vi "Terminal_Gear_System_Dispaly.vi"   [LabVIEW 2014]
types:
  T1 = cluster{"润滑油流量":u16, "油箱润滑油液位":u16, "油箱温度":u16, "冷却装置工作状态":u16, "供油压力":u16, "过滤器压差":u16, "油箱液位":u16, "供油油温":u16, "齿轮箱轴承温度":u16, "齿轮箱高速端输出转速":u16, "齿轮子系统状态字":cluster{"加热装置异常报警":bool, "冷却装置异常报警":bool, "油箱液位过低报警":bool, "供油油温过高报警":bool, "循环回路过滤器压差过高报警":bool, "1号油泵故障报警":bool, "2号油泵故障报警":bool, "供油压力过低报警":bool, "供油流量过低报警":bool, "轴承温度异常报警":bool, "油箱液位过高报警":bool, "回油过滤器压差过高报警":bool, "供油过滤器压差过高报警":bool}}
  T2 = cluster{"加热装置异常报警":bool, "冷却装置异常报警":bool, "油箱液位过低报警":bool, "供油油温过高报警":bool, "循环回路过滤器压差过高报警":bool, "1号油泵故障报警":bool, "2号油泵故障报警":bool, "供油压力过低报警":bool, "供油流量过低报警":bool, "轴承温度异常报警":bool, "油箱液位过高报警":bool, "回油过滤器压差过高报警":bool, "供油过滤器压差过高报警":bool}
  T3 = cluster{cluster{sgl, sgl, "润滑油流量":u16}, cluster{sgl, sgl, "油箱润滑油液位":u16}, cluster{sgl, sgl, "油箱温度":u16}, "冷却装置工作状态":u16, cluster{sgl, sgl, "供油压力":u16}, cluster{sgl, sgl, "过滤器压差":u16}, cluster{sgl, sgl, "油箱液位":u16}, cluster{sgl, sgl, "供油油温":u16}, cluster{sgl, sgl, "齿轮箱轴承温度":u16}, cluster{sgl, sgl, "齿轮箱高速端输出转速":u16}, "齿轮子系统状态字":cluster{"加热装置异常报警":bool, "冷却装置异常报警":bool, "油箱液位过低报警":bool, "供油油温过高报警":bool, "循环回路过滤器压差过高报警":bool, "1号油泵故障报警":bool, "2号油泵故障报警":bool, "供油压力过低报警":bool, "供油流量过低报警":bool, "轴承温度异常报警":bool, "油箱液位过高报警":bool, "回油过滤器压差过高报警":bool, "供油过滤器压差过高报警":bool}}
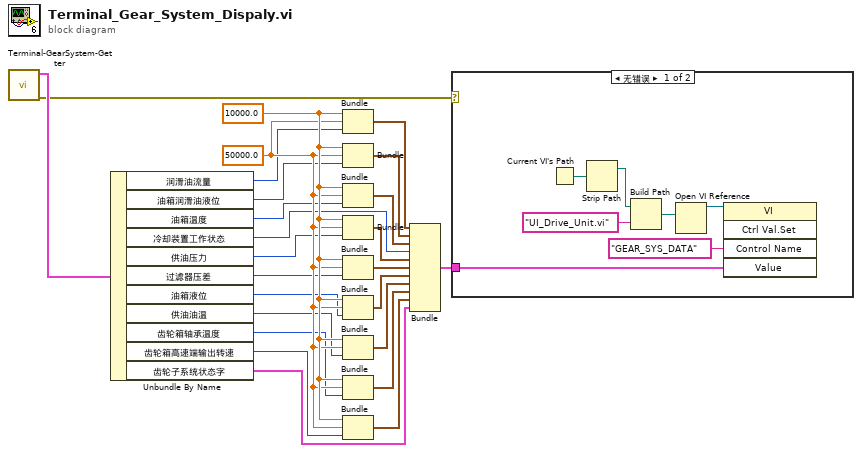
[diagram p0: block diagram]
diagram:
  w23 = sgl 50000.0
  w24 = sgl 10000.0
  n1 = call "Terminal-GearSystem-Getter.vi"() -> ("error out"=w2:errorcluster, "设备信息"=w25:T1)  [unwired: 10 in]
  n2 = Unbundle By Name(w25) -> ("润滑油流量"=w22:u16, "油箱润滑油液位"=w21:u16, "油箱温度"=w20:u16, "冷却装置工作状态"=w10:u16, "供油压力"=w19:u16, "过滤器压差"=w18:u16, "油箱液位"=w17:u16, "供油油温"=w16:u16, "齿轮箱轴承温度"=w15:u16, "齿轮箱高速端输出转速"=w14:u16, "齿轮子系统状态字"=w3:T2)
  n3 = Bundle(w24, w23, "润滑油流量"=w22) -> (w13:cluster{sgl, sgl, "润滑油流量":u16})  [unwired: 1 in]
  n4 = Bundle(w24, w23, "油箱润滑油液位"=w21) -> (w12:cluster{sgl, sgl, "油箱润滑油液位":u16})  [unwired: 1 in]
  n5 = Bundle(w24, w23, "油箱温度"=w20) -> (w11:cluster{sgl, sgl, "油箱温度":u16})  [unwired: 1 in]
  n6 = Bundle(w24, w23, "供油压力"=w19) -> (w9:cluster{sgl, sgl, "供油压力":u16})  [unwired: 1 in]
  n7 = Bundle(w24, w23, "过滤器压差"=w18) -> (w8:cluster{sgl, sgl, "过滤器压差":u16})  [unwired: 1 in]
  n8 = Bundle(w24, w23, "油箱液位"=w17) -> (w7:cluster{sgl, sgl, "油箱液位":u16})  [unwired: 1 in]
  n9 = Bundle(w24, w23, "供油油温"=w16) -> (w6:cluster{sgl, sgl, "供油油温":u16})  [unwired: 1 in]
  n10 = Bundle(w24, w23, "齿轮箱轴承温度"=w15) -> (w5:cluster{sgl, sgl, "齿轮箱轴承温度":u16})  [unwired: 1 in]
  n11 = Bundle(w24, w23, "齿轮箱高速端输出转速"=w14) -> (w4:cluster{sgl, sgl, "齿轮箱高速端输出转速":u16})  [unwired: 1 in]
  n12 = Bundle(w13, w12, w11, "冷却装置工作状态"=w10, w9, w8, w7, w6, w5, w4, "齿轮子系统状态字"=w3) -> (w1:T3)  [unwired: 1 in]
  n13 = case shown="无错误" w2 {
    tunnel: w1 -> [w26 _]
    frame No Error {
      n14 = Current VI's Path() -> (path=w30:path)
      n15 = Strip Path(path=w30) -> (stripped path=w31:path)  [unwired: 1 out]
      n16 = Build Path(base path=w31, name or relative path="UI_Drive_Unit.vi") -> (appended path=w28:path)
      n17 = Open VI Reference(vi path=w28) -> (vi reference=w27:refnum<vi>)  [unwired: 5 in, 1 out]
      n18 = invoke class="VI" method="Ctrl Val.Set"(reference=w27, "Control Name"="GEAR_SYS_DATA", "Value"=w26) -> ()  [unwired: 2 in, 5 out]
    }
    frame Error {
    }
  }
